vi "whileloop1.vi"() -> ()   [LabVIEW 2021]
panel:
  out "Numeric":i32
  in  "Stop":bool
  out "Iteration":i32
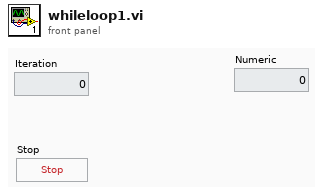
[diagram p1: front panel]
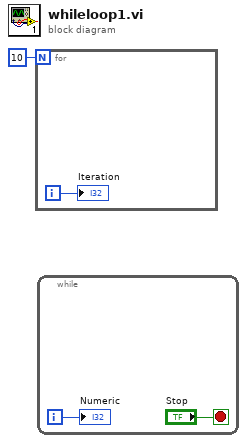
[diagram p0: block diagram]
diagram:
  n1 = for {
    N: 10 -> [_]
    i -> [w2]
    "Iteration" <- w2
  }
  n2 = while {
    i -> [w3]
    stop <- "Stop" stop-if-true
    "Numeric" <- w3
  }
